vi "Revision Query.vi"(8 "error in (no error)":errorcluster, 11 "VISA resource name":refnum<visa-resource-name>) -> (0 "error out":errorcluster, 1 "Instrument Firmware Revision":string, 2 "Instrument Driver Revision":string, 3 "VISA resource name out":refnum<visa-resource-name>)   [LabVIEW 2025, in "NewtonsPSM1735.lvlib"]
doc: "Queries the current instrument firmware revision and instrument driver revision.\n\nRefer to the Readme file for detailed driver information including modification history."
uses:
  NewtonsPSM1735.lvlib
panel:
  out "Instrument Serial Number":string
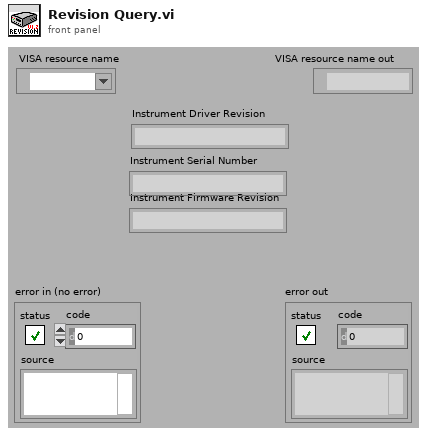
[diagram p1: front panel]
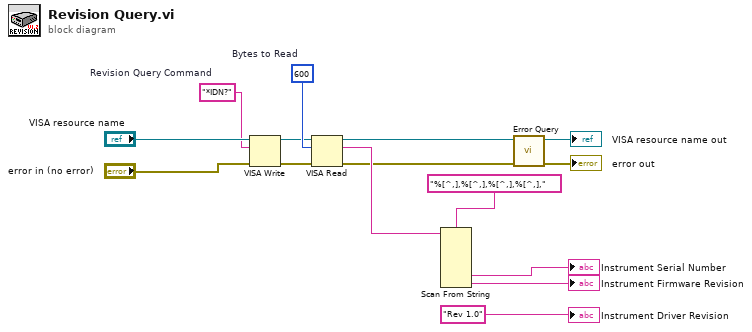
[diagram p0: block diagram]
diagram:
  w11 = "*IDN?"  # Revision Query Command
  w14 = u32 600  # Bytes to Read
  n1 = VISA Write(VISA resource name="VISA resource name", write buffer=w11, error in (no error)="error in (no error)") -> (VISA resource name out=w13:refnum<visa-resource-name>, error out=w12:errorcluster)  [unwired: 1 out]
  n2 = VISA Read(VISA resource name=w13, byte count=w14, error in (no error)=w12) -> (VISA resource name out=w7:refnum<visa-resource-name>, read buffer=w10:string, error out=w8:errorcluster)  [unwired: 1 out]
  n3 = Scan From String(format string="%[^,],%[^,],%[^,],%[^,],", input string=w10) -> (output 3=→"Instrument Serial Number":string, output 4=→"Instrument Firmware Revision":string)  [unwired: 2 in, 9 out]
  n4 = call "Error Query.vi"("error in (no error)"=w8, "VISA resource name"=w7) -> ("error out"=→"error out":errorcluster, "VISA resource name out"=→"VISA resource name out":refnum<visa-resource-name>)  [unwired: 8 out]
  "Instrument Driver Revision" <- "Rev 1.0"
